vi "Check for Input.vi"(8 "error in (no error)":errorcluster, 9 "Control Refs":refnum<vi>[](array[refnum]), 10 "Mouse Ref":refnum<k1>, 11 "Image Assertion in":refnum<class "Image Assertion.lvclass">) -> (0 "error out":errorcluster, 3 "Image Assertion out":refnum<class "Image Assertion.lvclass">)   [LabVIEW 2020, in "MacroAssert.lvlib" / "Image Assertion.lvclass"]
uses:
  Image Assertion.lvclass
  Image Assertion.lvclass/Image Assertion.ctl
  MacroAssert.lvlib
  <vilib>/Utility/inputDevices.llb/mouseAcquire.vi
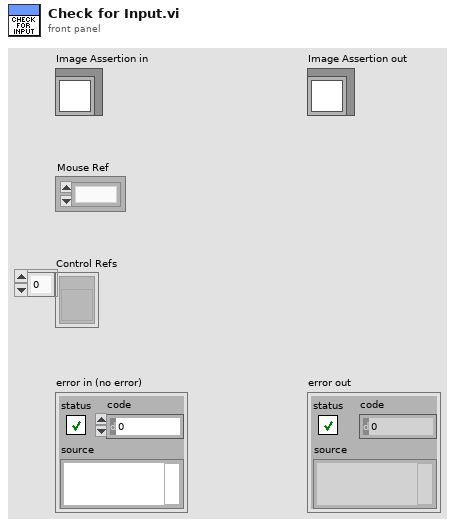
[diagram p1: front panel]
types:
  T1 = cluster{"button 1":bool, "button 2":bool, "button 3":bool, "button 4":bool}
  T2 = cluster{"left":i16, "top":i16, "right":i16, "bottom":i16}
  T3 = typedef "imagedata.ctl" = cluster{"image type":i32, "image depth":i32, "image":u8[], "mask":u8[], "colors":u32[], "Rectangle":cluster{"left":i16, "top":i16, "right":i16, "bottom":i16}}
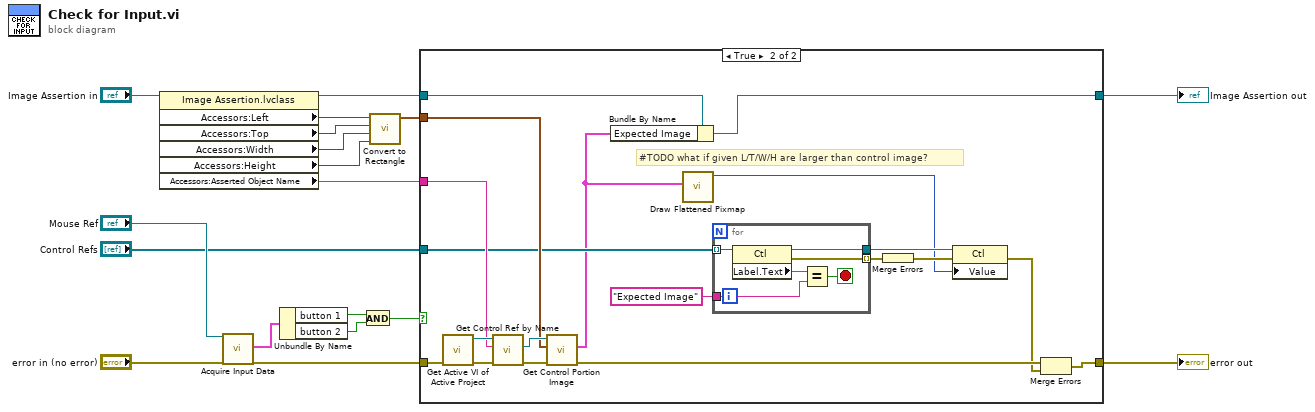
[diagram p0: block diagram]
diagram:
  n1 = property class="Image Assertion.lvclass"(reference="Image Assertion in") -> (reference out=w9:refnum<class "Image Assertion.lvclass">, "Accessors:Left"=w8:i16, "Accessors:Top"=w7:i16, "Accessors:Width"=w6:i16, "Accessors:Height"=w5:i16, "Accessors:Asserted Object Name"=w4:string)  [unwired: 1 in, 1 out]
  n2 = call-poly <vilib>:"Acquire Input Data.vi"("device ID"="Mouse Ref", "error in (no error)"="error in (no error)") -> ("button info"=w14:T1, "error out"=w15:errorcluster)  [unwired: 14 in, 2 out]
  n3 = Unbundle By Name(w14) -> ("button 1"=w12:bool, "button 2"=w13:bool)
  n4 = And(x=w12, y=w13) -> (x .and. y?=w11:bool)
  n5 = call "Convert to Rectangle.vi"("Height"=w5, "Width"=w6, "Top"=w7, "Left"=w8) -> ("Rectangle"=w10:T2)  [unwired: 7 in]
  n6 = case shown="True" w11 {
    tunnel: w9 -> [w19 w34]
    tunnel: [w19 w30] -> w2
    tunnel: w4 -> [_ w33]
    tunnel: w10 -> [_ w31]
    tunnel: w15 -> [w20 w37]
    tunnel: [w20 w22] -> w17
    tunnel: "Control Refs" -> [_ w27]
    frame False {
    }
    frame True {
      # "#TODO what if given L/T/W/H are larger than control image?"
      n7 = call "Get Active VI of Active Project.vi"("error in (no error)"=w37) -> ("error out"=w39:errorcluster, "Active VI Ref"=w35:refnum<vi>)  [unwired: 9 in]
      n8 = call "Get Control Ref by Name.vi"("error in (no error)"=w39, "Name"=w33, "VI Ref"=w35) -> ("error out"=w38:errorcluster, "Ctl Ref"=w32:refnum<vi>)  [unwired: 6 in, 1 out]
      n9 = call "Get Control Portion Image.vi"("error in (no error)"=w38, "subset rect"=w31, "Ctl Ref"=w32) -> ("error out"=w36:errorcluster, "Ctl Portion Image Data"=w26:T3)  [unwired: 6 in, 1 out]
      n10 = Bundle By Name(cluster=w34, "Expected Image"=w26) -> (w30:refnum<class "Image Assertion.lvclass">)
      n11 = call <vilib>:"Draw Flattened Pixmap.vi"("image data"=w26) -> ("new picture"=w23:picture)  [unwired: 8 in]
      n12 = for {
        tunnel: w27 -> [w45] mode=indexing
        tunnel: [w44] -> w25
        tunnel: "Expected Image" -> [w41]
        tunnel: [w40] -> w28 mode=indexing
        stop <- w42 stop-if-true
        n13 = property class="Ctl"(reference=w45) -> (reference out=w44:refnum<vi>, error out=w40:errorcluster, "Label.Text"=w43:string)  [unwired: 1 in]
        n14 = Equal?(x=w43, y=w41) -> (x = y?=w42:bool)
      }
      n15 = Merge Errors(w28) -> (w24:errorcluster)
      n16 = property class="Ctl"(reference=w25, error in=w24, "Value"=w23) -> (error out=w21:errorcluster)  [unwired: 1 out]
      n17 = Merge Errors(w36, w21) -> (w22:errorcluster)
    }
  }
  "error out" <- w17
  "Image Assertion out" <- w2
